vi "dNET_SQL_Bckup.vi"(4 "Bckup_DB?":bool, 6 "Table Data":bool=TRUE, 8 "error in (no error)":errorcluster, 11 "Table_Schema":path) -> (0 "error out":errorcluster)   [LabVIEW 2020]
uses:
  Microsoft.SqlServer.Smo
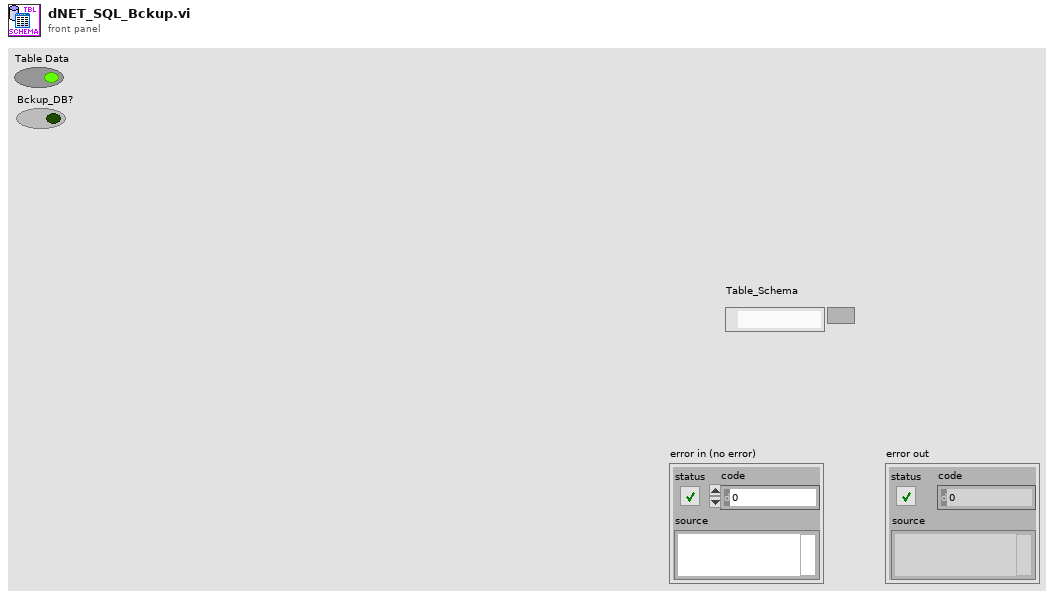
[diagram p1: front panel]
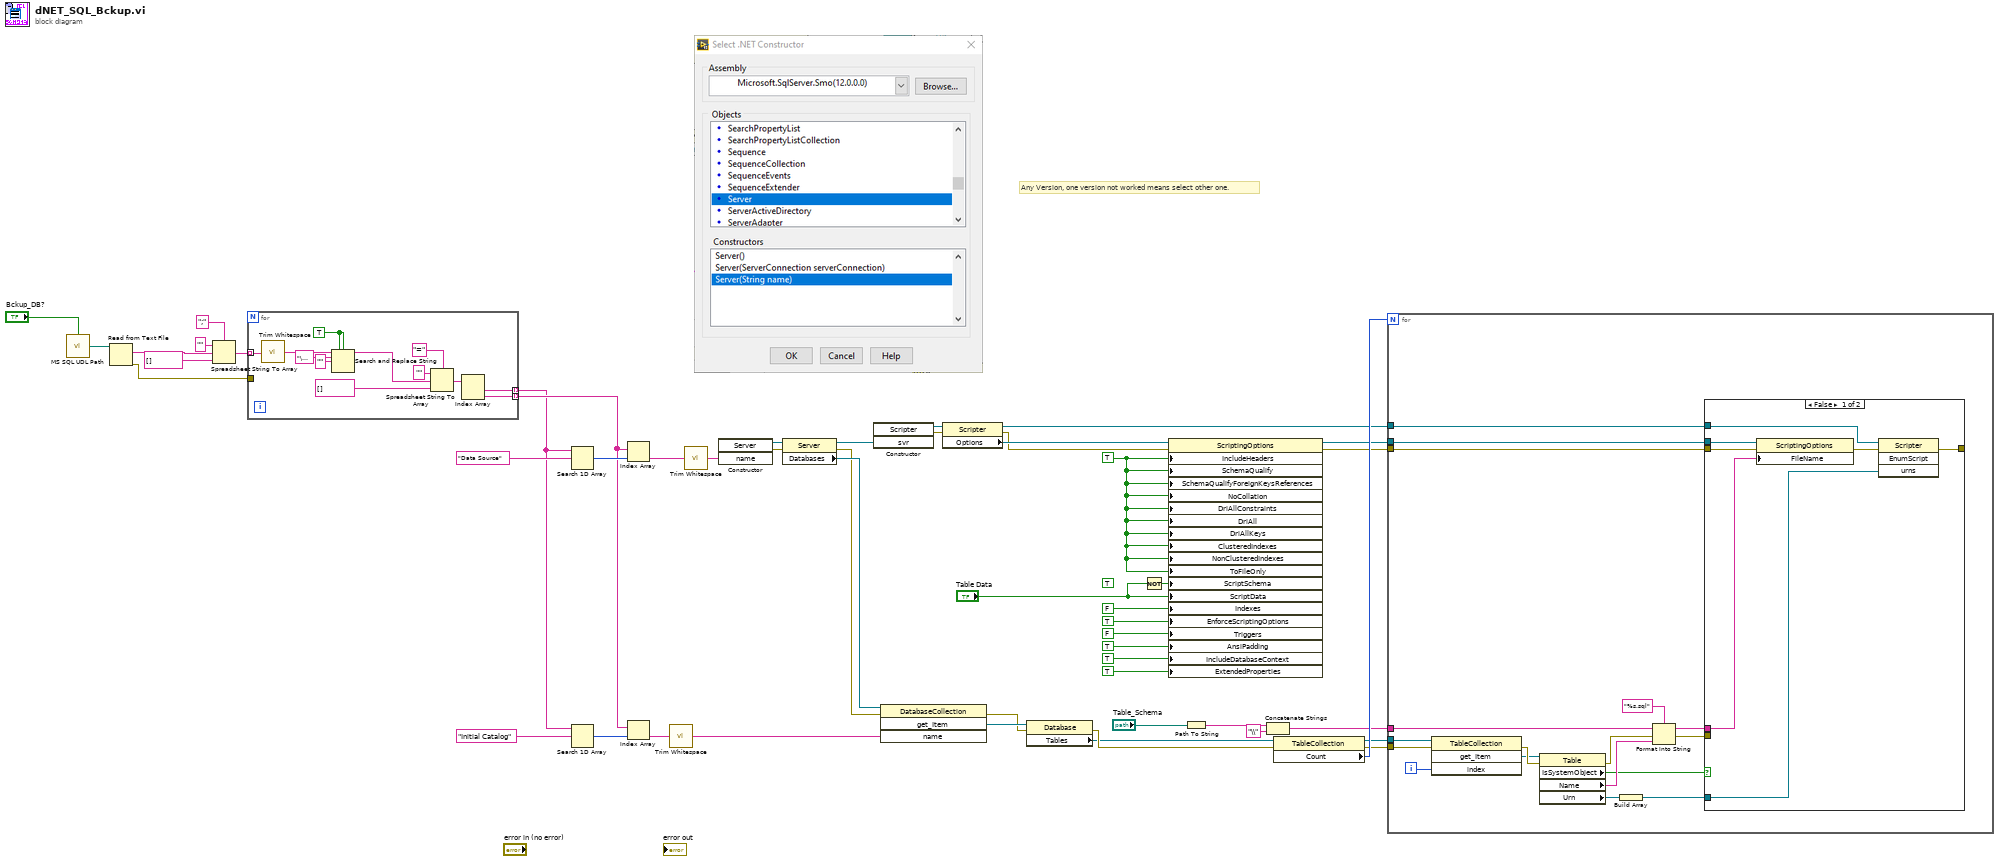
[diagram p0: block diagram]
diagram:
  (unwired) TRUE ("ScriptSchema")
  w9 = TRUE ("IncludeHeaders")
  # "Any Version, one version not worked means select other one."
  n1 = call "MS SQL UDL Path.vi"("Bckup_DB?"="Bckup_DB?") -> ("UDL File Location"=w33:path)  [unwired: 3 in]
  n2 = Read from Text File(file (use dialog)=w33) -> (text=w32:string, error out=w10:errorcluster)  [unwired: 3 in, 2 out]
  n3 = Spreadsheet String To Array(delimiter (Tab)=";", format string="", spreadsheet string=w32, array type (2D Dbl)=string[] []) -> (array=w28:string[])
  n4 = for {
    tunnel: w28 -> [w62] mode=indexing
    tunnel: [w52] -> w20 mode=indexing
    tunnel: [w51] -> w23 mode=indexing
    tunnel: w10 -> [_]
    w58 = TRUE ("replace all? (F)")
    n5 = call <vilib>:"Trim Whitespace.vi"("string"=w62) -> ("trimmed string"=w61:string)  [unwired: 1 in]
    n6 = Search and Replace String(replace all?=w58, case sensitive?=w58, input string=w61, search string="\u0000", replace string="" ("replace string (\"\")")) -> (result string=w54:string)  [unwired: 3 in, 3 out]
    n7 = Spreadsheet String To Array(delimiter (Tab)="=", format string="", spreadsheet string=w54, array type (2D Dbl)=string[] []) -> (array=w53:string[])
    n8 = Index Array(array=w53) -> (element #1=w52:string, element #2=w51:string)  [unwired: 2 in]
  }
  n9 = Search 1D Array(1D array=w20, element="Data Source" ("name 2")) -> (index of element=w24:i32)  [unwired: 1 in]
  n10 = Search 1D Array(1D array=w20, element="Initial Catalog" ("name")) -> (index of element=w25:i32)  [unwired: 1 in]
  n11 = Index Array(array=w23, index=w24) -> (element=w22:string)
  n12 = Index Array(array=w23, index=w25) -> (element=w21:string)
  n13 = call <vilib>:"Trim Whitespace.vi"("string"=w21) -> ("trimmed string"=w19:string)  [unwired: 1 in]
  n14 = call <vilib>:"Trim Whitespace.vi"("string"=w22) -> ("trimmed string"=w13:string)  [unwired: 1 in]
  n15 = constructor class="Server"("name"=w13) -> (reference out=w1:refnum<k24>, error out=w50:errorcluster)  [unwired: 3 in, 2 out]
  n16 = property class="Server"(reference=w1, error in=w50) -> (reference out=w47:refnum<k24>, error out=w48:errorcluster, "Databases"=w49:refnum<k24>)
  n17 = constructor class="Scripter"("svr"=w47) -> (reference out=w46:refnum<k24>, error out=w45:errorcluster)  [unwired: 3 in, 2 out]
  n18 = invoke class="DatabaseCollection" method="get_Item"(reference=w49, error in=w48, "name"=w19) -> (error out=w37:errorcluster, "get_Item"=w38:refnum<k24>)  [unwired: 1 in, 2 out]
  n19 = property class="Scripter"(reference=w46, error in=w45) -> (reference out=w35:refnum<k24>, error out=w43:errorcluster, "Options"=w44:refnum<k24>)
  n20 = property class="Database"(reference=w38, error in=w37) -> (error out=w34:errorcluster, "Tables"=w14:refnum<k24>)  [unwired: 1 out]
  n21 = Not(x="Table Data") -> (.not. x?=w2:bool)
  n22 = property class="ScriptingOptions"(reference=w44, error in=w43, "IncludeHeaders"=w9, "SchemaQualify"=w9, "SchemaQualifyForeignKeysReferences"=w9, "NoCollation"=w9, "DriAllConstraints"=w9, "DriAll"=w9, "DriAllKeys"=w9, "ClusteredIndexes"=w9, "NonClusteredIndexes"=w9, "ToFileOnly"=w9, "ScriptSchema"=w2, "ScriptData"="Table Data", "Indexes"=FALSE, "EnforceScriptingOptions"=TRUE, "Triggers"=FALSE, "AnsiPadding"=TRUE, "IncludeDatabaseContext"=TRUE, "ExtendedProperties"=TRUE) -> (reference out=w36:refnum<k24>, error out=w39:errorcluster)
  n23 = Path To String(path="Table_Schema") -> (string=w17:string)
  n24 = Concatenate Strings(w17, "\\" ("string")) -> (w16:string)
  n25 = property class="TableCollection"(reference=w14, error in=w34) -> (reference out=w40:refnum<k24>, error out=w41:errorcluster, "Count"=w42:i32)
  n26 = for {
    N: w42 -> [_]
    tunnel: w41 -> [w64]
    tunnel: w40 -> [w79]
    tunnel: w39 -> [w70]
    tunnel: w36 -> [w76]
    tunnel: w35 -> [w72]
    tunnel: w16 -> [w67]
    i -> [w78]
    n27 = invoke class="TableCollection" method="get_Item"(reference=w79, error in=w64, "index"=w78) -> (error out=w77:errorcluster, "get_Item"=w65:refnum<k24>)  [unwired: 1 in, 2 out]
    n28 = property class="Table"(reference=w65, error in=w77) -> (error out=w63:errorcluster, "IsSystemObject"=w69:bool, "Name"=w75:string, "Urn"=w66:refnum<k24>)  [unwired: 1 out]
    n29 = Build Array(w66) -> (w71:refnum<k24>[])
    n30 = Format Into String(format string="%s.sql" ("FileName"), initial string=w67, error in=w63, w75) -> (resulting string=w73:string, error out=w68:errorcluster)
    n31 = case shown="False" w69 {
      tunnel: w76 -> [w86 _]
      tunnel: w73 -> [w85 _]
      tunnel: w72 -> [w84 _]
      tunnel: w71 -> [w82 _]
      tunnel: w70 -> [w81 _]
      tunnel: w68 -> [_ _]
      tunnel: [w80 _] -> _
      frame False {
        n32 = property class="ScriptingOptions"(reference=w86, error in=w81, "FileName"=w85) -> (error out=w83:errorcluster)  [unwired: 1 out]
        n33 = invoke class="Scripter" method="EnumScript"(reference=w84, error in=w83, "urns"=w82) -> (error out=w80:errorcluster)  [unwired: 1 in, 3 out]
      }
      frame True {
      }
    }
  }
